vi "Stop Response Complete.vi"(8 "error in (no error)":errorcluster, 11 "Pulse Controller in":refnum<class "Pulse Controller.lvclass">) -> (0 "error out":errorcluster, 3 "Pulse Controller out":refnum<class "Pulse Controller.lvclass">)   [LabVIEW 2021, in "Pulse Controller.lvclass"]
uses:
  Pulse Controller.lvclass
  Pulse Controller.lvclass/Pulse Controller.ctl
  Process Controller Messages/Start Measurements Msg/Start Measurements Msg.lvclass
  <vilib>/ActorFramework/Actor/Actor.lvclass
  Process Controller/Request type.ctl
  Process Controller/Process Controller.lvclass
  C:/Program Files/National Instruments/LabVIEW 2021/vi.lib/ActorFramework/Actor/Actor.lvclass
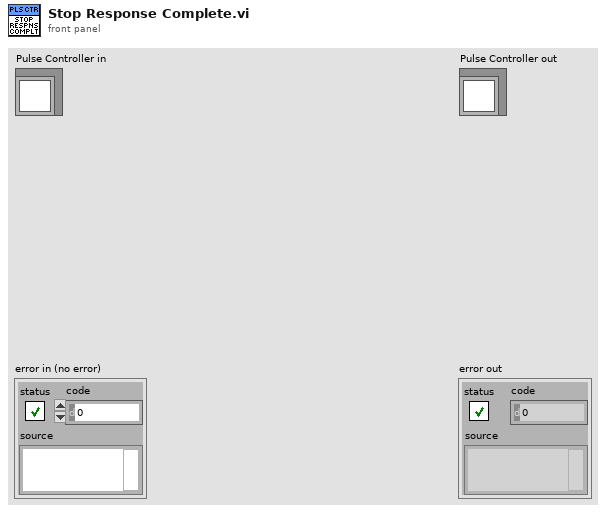
[diagram p1: front panel]
types:
  T1 = typedef "Request type.ctl" = enum16{"Process complete", "User command", "Auto-restart", "Error"}
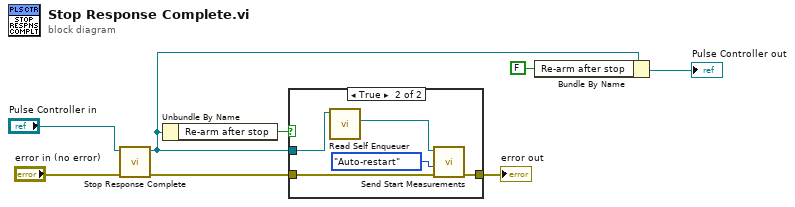
[diagram p0: block diagram]
diagram:
  n1 = call-parent "Stop Response Complete.vi"("error in (no error)"="error in (no error)", "Process Controller in"="Pulse Controller in") -> ("error out"=w6:errorcluster, "Process Controller out"=w4:refnum<class "Pulse Controller.lvclass">)  [unwired: 8 in]
  n2 = Unbundle By Name(w4) -> ("Re-arm after stop"=w3:bool)
  n3 = case shown="True" w3 {
    tunnel: w6 -> [w9 w14]
    tunnel: [w9 w13] -> w5
    tunnel: w4 -> [_ w10]
    frame False {
    }
    frame True {
      n4 = call <vilib>:"Read Self Enqueuer.vi"("Actor"=w10) -> ("Self Enqueuer"=w12:refnum<class "Message Enqueuer.lvclass">)  [unwired: 10 in]
      n5 = call "Send Start Measurements.vi"("error in (no error)"=w14, "Request type"=Request_type."Auto-restart", "Message Enqueuer"=w12) -> ("error out"=w13:errorcluster)  [unwired: 7 in, 1 out]
    }
  }
  "error out" <- w5
  n6 = Bundle By Name(cluster=w4, "Re-arm after stop"=FALSE) -> (→"Pulse Controller out":refnum<class "Pulse Controller.lvclass">)
